vi "RT main.vi"() -> ()   [LabVIEW 2017]
doc: "This example demonstrates how to acquire a continuous amount of data (Waveform) using the DAQ device's internal clock. It also shows how to synchronize two devices for different device families (E Series, S Series, M Series, X Series, DSA, and SC Express), to simultaneously acquire the data.\n\nFor instructions on how to connect your signals to the DAQ device, refer to your device documentation."
uses:
  <vilib>/addons/_NISVFA/_Shared subVIs/Controls/svc_Engineering Units Text Ring.ctl
  <vilib>/addons/_NISVFA/_Shared subVIs/Controls/svc_Weighting Filter Text Ring.ctl
  typedefs/Data.ctl
  <vilib>/Utility/error.llb/DialogType.ctl
  <vilib>/DAQmx/read.llb/DAQmx Read (Analog 1D Wfm NChan NSamp).vi
  <vilib>/Analysis/baseanly.llb/Mean (DBL).vi
  <vilib>/DAQmx/read.llb/DAQmx Read (Analog Wfm 1Chan NSamp).vi
  <vilib>/addons/Sound and Vibration/svt_Calibration/SVL Scale Voltage to EU (1 Ch).vi
  <vilib>/DAQmx/read.llb/DAQmx Read (Analog DBL 1Chan 1Samp).vi
  <vilib>/addons/_NISVFA/_Shared subVIs/Common/svc_Set SV Channel Info.vi
  <vilib>/addons/_NISVFA/_Shared subVIs/Common/svc_Set SV Channel Info (variant).vi
  <vilib>/addons/_NISVFA/_Shared subVIs/Common/SVL Set dB Reference (variant).vi
  <vilib>/DAQmx/create/channels.llb/DAQmx Create Channel (AI-Voltage-Basic).vi
  <vilib>/DAQmx/configure/timing.llb/DAQmx Timing (Sample Clock).vi
  <vilib>/DAQmx/create/channels.llb/DAQmx Create Channel (AI-Temperature-Thermocouple).vi
  <vilib>/httpClient/POSTBuffer.vi
  <vilib>/DAQmx/miscellaneous.llb/DAQmx Fill In Error Info.vi
  <vilib>/addons/Sound and Vibration/Order Analysis/Tach Process/OAT Analog Tacho Process (1 Tacho).vi
  <vilib>/addons/_NISVFA/_Shared subVIs/Common/svc_Engineering Units to Unit Label.vi
  <vilib>/addons/_NISVFA/_Shared subVIs/Common/svc_Compute Scale Factor to Convert V to EU.vi
  <vilib>/addons/_NISVFA/_Shared subVIs/Common/svc_Compute Scale Factor to Convert C to EU.vi
  <vilib>/addons/_NISVFA/_Shared subVIs/Common/svc_Set dB ref if Pascal.vi
  <vilib>/addons/_NISVFA/_Shared subVIs/Common/svc_Caller VI Returned in Error Source.vi
  <vilib>/addons/Sound and Vibration/svt_Level/SVL Running RMS Level (1 Ch).vi
  <vilib>/addons/Sound and Vibration/svt_Calibration/SoundVib_Calibration.lvlib
  <vilib>/addons/Sound and Vibration/svt_Level/SoundVib_VibrationLevel.lvlib
  <vilib>/addons/Sound and Vibration/Order Analysis/Tach Process/SoundVib_TachProcess.lvlib
  <vilib>/Analysis/NI_AALBase.lvlib
  <vilib>/httpClient/LabVIEWHTTPClient.lvlib
  <vilib>/NI_Real-Time Target Support.lvlib
panel:
  out "dequeue elements":T1 {"RMS" format="%0.6f"; "RPM" format="%0.2f"; "Voltage" format="%0.2f"; "Current" format="%0.2f"; "Temperature" format="%0.2f"}
  out "flush elements":T1[](array[typedef]) {"RMS" format="%0.2f"; "RPM" format="%0.2f"; "Voltage" format="%0.2f"; "Current" format="%0.2f"; "Temperature" format="%0.2f"}
  out "Y":bool
  out "Numeric 2":i32
  out "Numeric":i32
  out "# elements in queue":i32
  in  "DIO STOP":bool
  in  "Buttoon 1":bool
  in  "Button 2":bool
  in  "Button 3":bool
  in  "Ipad 2":bool
  in  "Ipad 3":bool
  in  "Ipad 1":bool
  out "Valve":bool[](array[boolean])
  in  "Web server LED":bool
  out "X":bool
  out "JSON":string
  in  "integration time [s]":dbl=1.0
  out "Temp.":dbl format="%0.2f"
  out "Current":dbl format="%0.2f"
  out "Voltage":dbl format="%0.2f"
  out "RPM mean":dbl format="%0.2f"
  out "Motor Voltage & Current":waveform(dbl)[](graph)
  in  "Vibration Channel Info":T4={"sensor sensitivity"=1000.0, "engineering units"=1, "dB reference"=1.0, "custom label"="EU", "weighting filter"=0, "pregain"=0.0} {"pregain" format="%.2f"; "weighting filter" items=["Linear", "A-weighting", "B-weighting", "C-weighting", "ITU-R 468-4", "Dolby", "CCITT", "C-message", "Wb", "Wc", "Wd", "We", "Wf", "Wh", "Wj", "Wk", "Wm", "AES17 20 kHz lowpass", "AES17 40 kHz lowpass", "AES17 20 kHz highpass", "AES17 40 kHz highpass"]; "dB reference" format="%^.1e"; "engineering units" items=["custom..."=0, "V"=1, "A"=21, "C"=30, "pC"=31, "s"=32, "-"=29, "Pa"=2, "N"=20, "g"=3, "m/s^2"=4, "m/s"=5, "m"=6, "mm/s"=12, "mm"=13, "micron/s"=14, "micron"=15, "in/s^2"=7, "in/s"=8, "in"=9, "mil/s"=10, "mil"=11, "rad/s^2"=16, "rad/s"=17, "rad"=18, "deg/s^2"=26, "deg/s"=27, "deg"=28, "RPM"=22, "cycle/s^2"=23, "Hz"=24, "cycle"=25, "strain"=19]; "sensor sensitivity" format="%#_5f"}
  out "running RMS":dbl caption="g rms" format="%0.6f"
  in  "Acquire Stop":bool
  in  "CJC Channel":refnum<k21>
  in  "CJC Value":dbl=25.0 format="%0.2f"
  in  "CJC Source":i32(ring)=10116 items=["Built-In"=10200, "Constant Value"=10116, "Channel"=10113]
  in  "Thermocouple Type":i32(ring)=10073 items=["J"=10072, "K"=10073, "N"=10077, "R"=10082, "S"=10085, "T"=10086, "B"=10047, "E"=10055]
  in  "Units":i32(ring)=10143 items=["Deg C"=10143, "Deg F"=10144, "Kelvins"=10325, "Deg R"=10145, "From Custom Scale"=10065]
  in  "Max Temperature":dbl=35.0
  in  "Min Temperature":dbl
  out "Thermocouple waveform":dbl(graph)
  in  "Thermocouple Sample":i32=1
  in  "Motor Voltage & \nCurrent & RPM Sample":i32=2560
  in  "Motor Voltage & Current & RPM Sample Rate":dbl=25600.0
  in  "Thermocouple":tag="Mod3/ai0"
  out "Vibration":waveform(dbl)(graph)
  in  "Vibration Sample":i32=2560
  in  "Vibration Sample Rate":dbl=25600.0
  in  "Motor Voltage &Current& RPM":tag="Mod2/ai0:2"
  in  "Vibration":tag="Mod1/ai0"
  # "Vibration Settings"
  # "Vibration"
  # "Motor Voltage & Current & RPM"
  # "Motor Voltage & current & RPM Settings"
  # "Temperature"
  # "Tempearture"
  # "Thermocouple Settings"
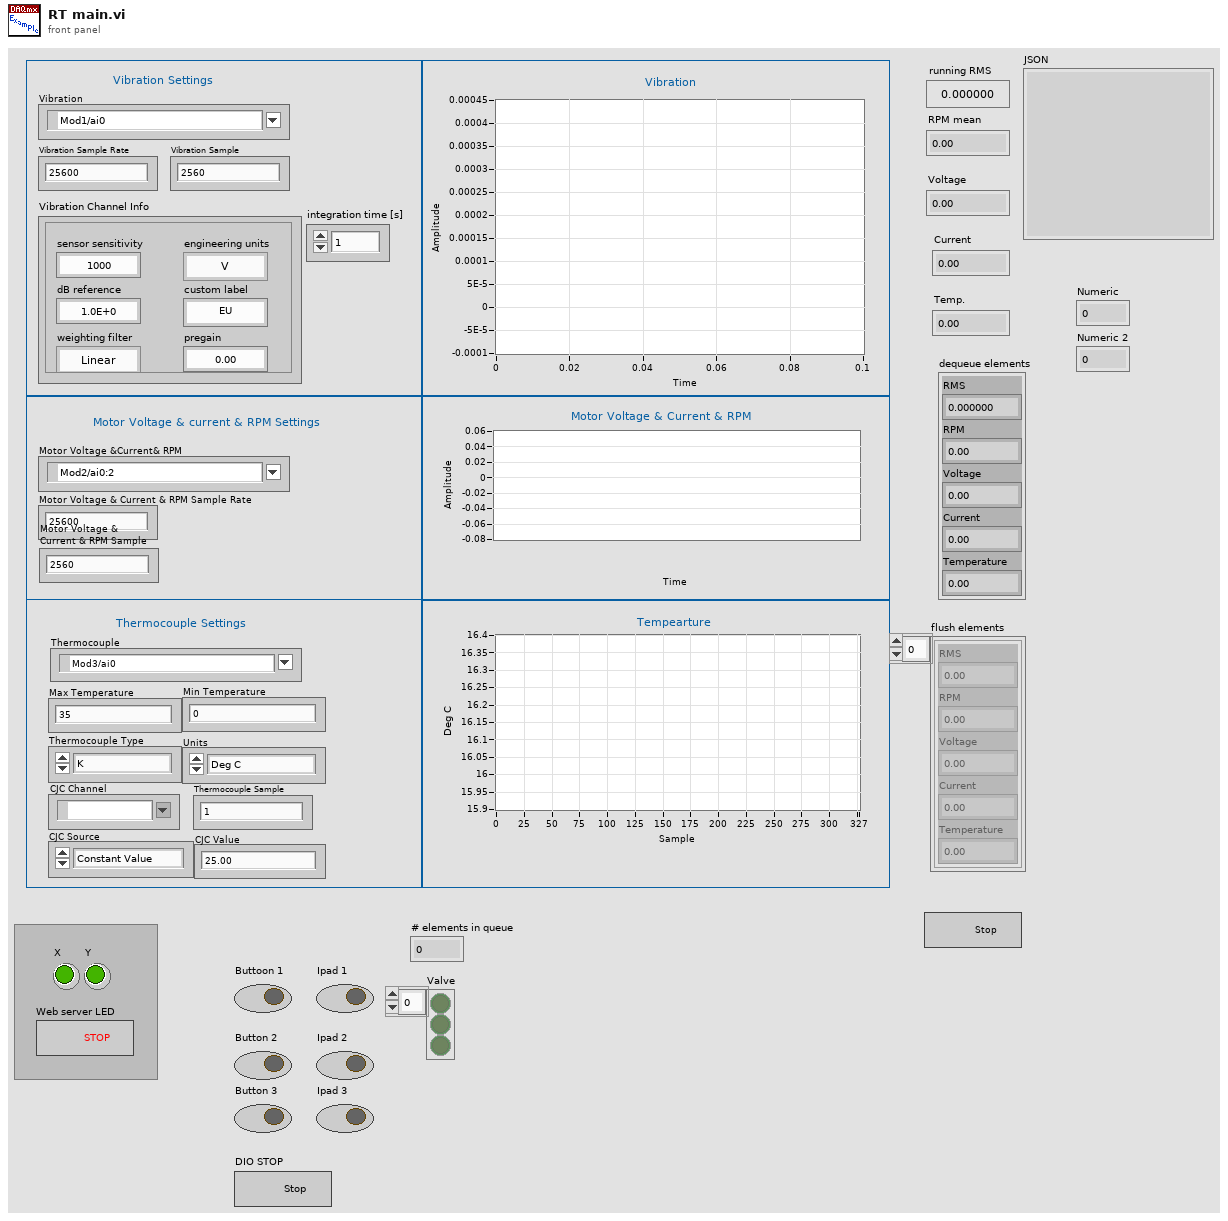
[diagram p1: front panel]
types:
  T1 = typedef "Data.ctl" = cluster{"RMS":dbl, "RPM":dbl, "Voltage":dbl, "Current":dbl, "Temperature":dbl}
  T2 = typedef "svc_Engineering Units Text Ring.ctl" = u16
  T3 = typedef "svc_Weighting Filter Text Ring.ctl" = u16
  T4 = cluster{"sensor sensitivity":dbl, "engineering units":T2, "dB reference":dbl, "custom label":string, "weighting filter":T3, "pregain":dbl}
  T5 = typedef "DialogType.ctl" = u16
  T6 = typedef "SoundVib_TachProcess.lvlib/speed profile.ctl" = cluster{"time [s]":dbl[], "speed [RPM]":dbl[]}
  T7 = typedef "LabVIEWHTTPClient.lvlib/ClientHandle.ctl" = refnum<k1>
  T8 = cluster{"RMS":dbl, "RPM":dbl, "Voltage":dbl, "Current":dbl, "Temperature":dbl}
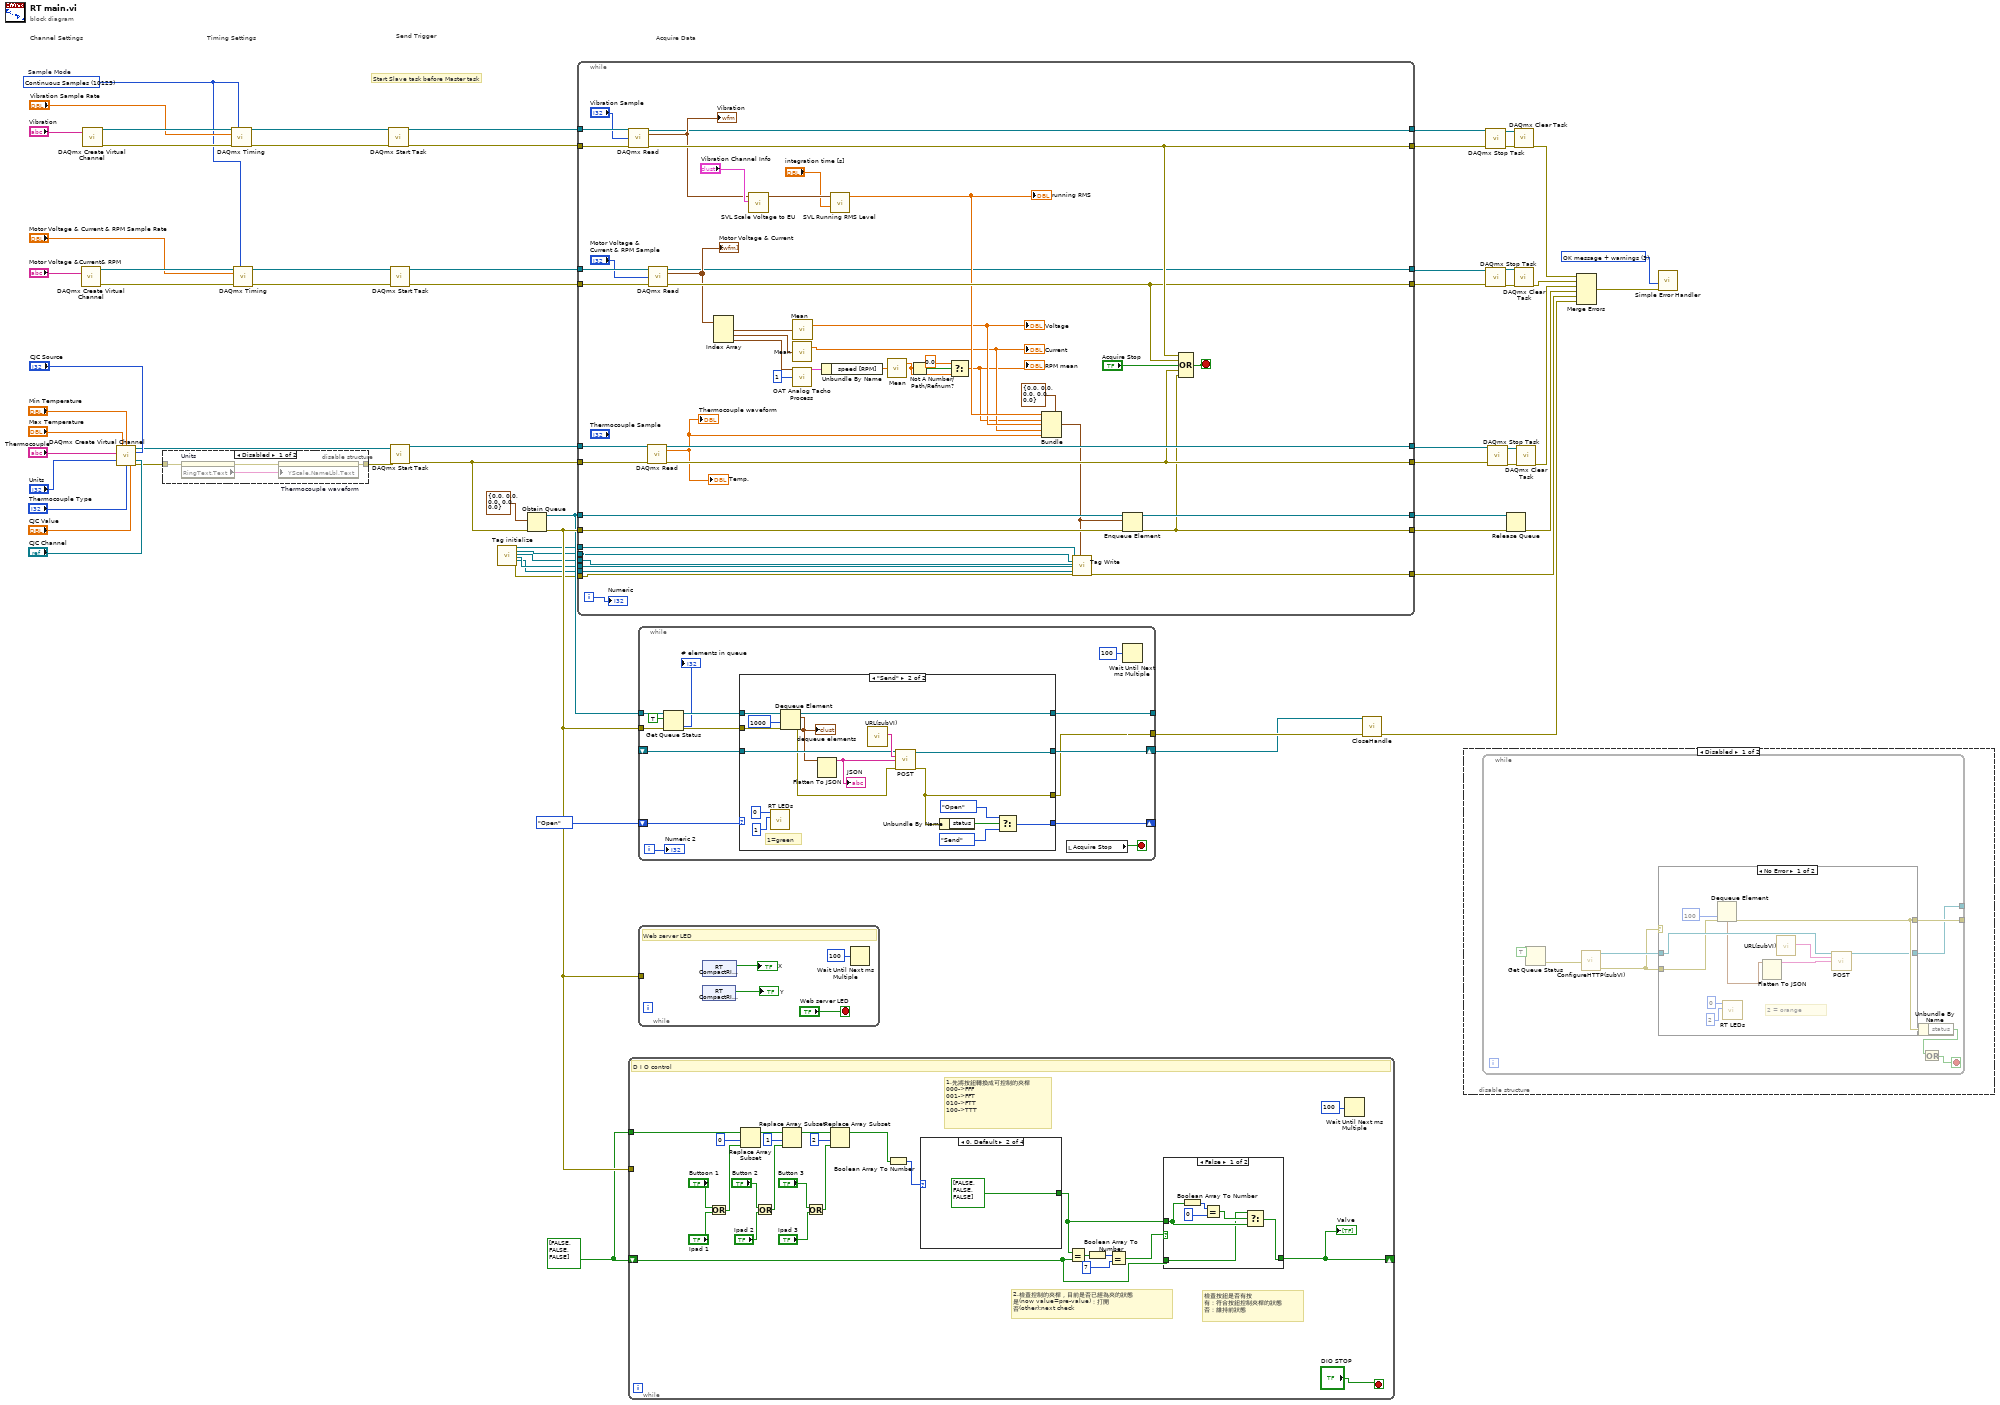
[diagram p0: block diagram]
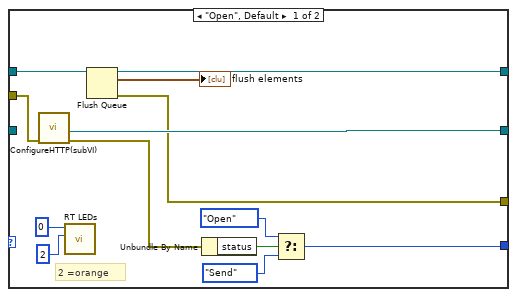
[diagram p3: hidden frame]
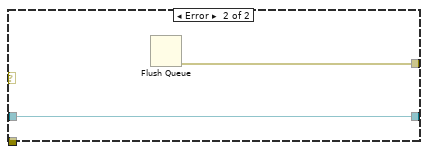
[diagram p4: hidden frame]
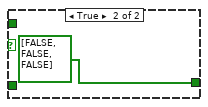
[diagram p6: hidden frame]
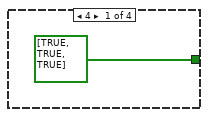
[diagram p7: hidden frame]
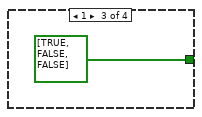
[diagram p8: hidden frame]
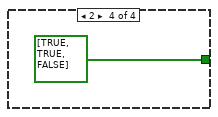
[diagram p9: hidden frame]
diagram:
  w9 = bool[] [FALSE, FALSE, FALSE]
  w41 = T5 3 items=["no dialog", "OK message", "continue or stop message", "OK message + warnings", "continue/stop + warnings"] ("type of dialog (OK msg:1)")
  w40 = 10123 items=["Finite Samples"=10178, "Continuous Samples"=10123, "Hardware Timed Single Point"=12522]  # Sample Mode
  # "Send Trigger"
  # "Acquire Data"
  # "Timing Settings"
  # "Channel Settings"
  # "Start Slave task before Master task"
  n1 = call-poly <vilib>:"DAQmx Create Virtual Channel.vi"("physical channels"="Motor Voltage &Current& RPM") -> ("task out"=w44:refnum<k21>, "error out"=w46:errorcluster)  [unwired: 13 in]
  n2 = call-poly <vilib>:"DAQmx Create Virtual Channel.vi"("physical channels"="Vibration") -> ("task out"=w48:refnum<k21>, "error out"=w47:errorcluster)  [unwired: 13 in]
  n3 = call-poly <vilib>:"DAQmx Create Virtual Channel.vi"("maximum value"="Max Temperature", "minimum value"="Min Temperature", "physical channels"="Thermocouple", "cjc source"="CJC Source", "units"="Units", "cjc channel"="CJC Channel", "thermocouple type"="Thermocouple Type", "cjc value"="CJC Value") -> ("task out"=w22:refnum<k21>, "error out"=w24:errorcluster)  [unwired: 6 in]
  n4 = disable-structure shown="Disabled" {
    disable-tunnel: w24 -> [w69 w70]
    disable-tunnel: [w66 w70] -> w21
    frame Disabled {
      n5 = property on="Units" class="Ring (strict)"(error in=w69) -> (error out=w67:errorcluster, "RingText.Text"=w68:string)  [unwired: 1 in, 1 out]
      n6 = property on="Thermocouple waveform" class="WFChart (strict)"(error in=w67, "YScale.NameLbl.Text"=w68) -> (error out=w66:errorcluster)  [unwired: 1 in, 1 out]
    }
    frame Enabled {
    }
  }
  n7 = call-poly <vilib>:"DAQmx Timing.vi"("task/channels in"=w48, "sample mode"=w40, "rate"="Vibration Sample Rate", "error in"=w47) -> ("task out"=w17:refnum<k21>, "error out"=w38:errorcluster)  [unwired: 10 in]
  n8 = call-poly <vilib>:"DAQmx Timing.vi"("task/channels in"=w44, "sample mode"=w40, "rate"="Motor Voltage & Current & RPM Sample Rate", "error in"=w46) -> ("task out"=w45:refnum<k21>, "error out"=w43:errorcluster)  [unwired: 10 in]
  n9 = call <vilib>:"DAQmx Start Task.vi"("task/channels in"=w17, "error in"=w38) -> ("task out"=w65:refnum<k21>, "error out"=w64:errorcluster)  [unwired: 12 in]
  n10 = call <vilib>:"DAQmx Start Task.vi"("task/channels in"=w45, "error in"=w43) -> ("task out"=w63:refnum<k21>, "error out"=w62:errorcluster)  [unwired: 12 in]
  n11 = call <vilib>:"DAQmx Start Task.vi"("task/channels in"=w22, "error in"=w21) -> ("task out"=w37:refnum<k21>, "error out"=w16:errorcluster)  [unwired: 12 in]
  n12 = call "Tag initialize.vi"() -> ("RMS tag"=w7:refnum<class "NI Skyline Tag.lvclass">, "RPM tag"=w6:refnum<class "NI Skyline Tag.lvclass">, "Voltage tag"=w5:refnum<class "NI Skyline Tag.lvclass">, "Current Tag"=w4:refnum<class "NI Skyline Tag.lvclass">, "Temper tag"=w3:refnum<class "NI Skyline Tag.lvclass">, "error out"=w2:errorcluster)  [unwired: 14 in]
  n13 = Obtain Queue(element data type=T1 {"RMS"=0.0, "RPM"=0.0, "Voltage"=0.0, "Current"=0.0, "Temperature"=0.0} ("Data"), error in (no error)=w16) -> (queue out=w12:refnum<queue>, error out=w13:errorcluster)  [unwired: 3 in, 1 out]
  n14 = while {
    tunnel: w37 -> [w111]
    tunnel: w16 -> [w110]
    tunnel: [w109] -> w34
    tunnel: [w108] -> w33
    tunnel: w12 -> [w99]
    tunnel: [w96] -> w20
    tunnel: [w95] -> w19
    tunnel: w13 -> [w94]
    tunnel: w65 -> [w118]
    tunnel: [w87] -> w61
    tunnel: w63 -> [w115]
    tunnel: [w88] -> w57
    tunnel: w62 -> [w114]
    tunnel: [w113] -> w56
    tunnel: w64 -> [w117]
    tunnel: [w116] -> w60
    tunnel: w7 -> [w77]
    tunnel: w6 -> [w76]
    tunnel: w5 -> [w75]
    tunnel: w4 -> [w74]
    tunnel: w3 -> [w73]
    tunnel: w2 -> [w72]
    tunnel: [w71] -> w1
    i -> [w86]
    stop <- w119 stop-if-true
    n15 = call-poly <vilib>:"DAQmx Read.vi"("task/channels in"=w118, "number of samples per channel"="Vibration Sample", "error in"=w117) -> ("task out"=w87:refnum<k21>, "data"=w90:waveform(dbl), "error out"=w116:errorcluster)  [unwired: 10 in]
    "Vibration" <- w90
    n16 = call-poly <vilib>:"DAQmx Read.vi"("task/channels in"=w111, "error in"=w110) -> ("task out"=w109:refnum<k21>, "data"=w93:dbl, "error out"=w108:errorcluster)  [unwired: 11 in]
    "Thermocouple waveform" <- w93
    "Temp." <- w93
    n17 = call-poly <vilib>:"DAQmx Read.vi"("task/channels in"=w115, "number of samples per channel"="Motor Voltage & \nCurrent & RPM Sample", "error in"=w114) -> ("task out"=w88:refnum<k21>, "data"=w101:waveform(dbl)[], "error out"=w113:errorcluster)  [unwired: 10 in]
    "Motor Voltage & Current" <- w101
    n18 = Index Array(array=w101) -> (element #1=w100:waveform(dbl), element #2=w92:waveform(dbl), element #3=w91:waveform(dbl))  [unwired: 3 in]
    n19 = call-poly <vilib>:"SVL Scale Voltage to EU.vi"("channel info"="Vibration Channel Info", "signal [V]"=w90) -> ("scaled signal [EU]"=w105:waveform(dbl))  [unwired: 7 in, 2 out]
    n20 = call-poly <vilib>:"Mean.vi"("X"=w92) -> ("mean"=w83:dbl)  [unwired: 1 out]
    "Current" <- w83
    n21 = call-poly <vilib>:"OAT Analog Tacho Process.vi"("analog tacho signal"=w91, "pulse/revolution (1)"=1) -> ("speed profile"=w103:T6)  [unwired: 9 in, 4 out]
    n22 = call-poly <vilib>:"Mean.vi"("X"=w100) -> ("mean"=w97:dbl)  [unwired: 1 out]
    "Voltage" <- w97
    n23 = Unbundle By Name(w103) -> ("speed [RPM]"=w102:dbl[])
    n24 = call-poly <vilib>:"SVL Running RMS Level.vi"("integration time [s]"="integration time [s]", "scaled signal [EU]"=w105) -> ("running RMS level [EU rms]"=w98:dbl)  [unwired: 6 in, 3 out]
    "running RMS" <- w98
    n25 = call-poly <vilib>:"Mean.vi"("X"=w102) -> ("mean"=w79:dbl)  [unwired: 1 out]
    n26 = Not A Number/Path/Refnum?(number/path/refnum=w79) -> (NaN/Path/Refnum?=w82:bool)
    n27 = Select(t=0.0, s=w82, f=w79) -> (s? t:f=w80:dbl)
    "RPM mean" <- w80
    n28 = Bundle(cluster=T1 {"RMS"=0.0, "RPM"=0.0, "Voltage"=0.0, "Current"=0.0, "Temperature"=0.0} ("Data"), "RMS"=w98, "RPM"=w80, "Voltage"=w97, "Current"=w83, "Temperature"=w93) -> (w78:T1)
    n29 = call "Tag Write.vi"("RMS tag"=w77, "RPM tag"=w76, "Voltage tag"=w75, "Current tag"=w74, "Temper tag"=w73, "error in (no error)"=w72, "Data"=w78) -> ("error out"=w71:errorcluster)  [unwired: 12 in]
    n30 = Enqueue Element(queue=w99, element=w78, error in (no error)=w94) -> (queue out=w96:refnum<queue>, error out=w95:errorcluster)  [unwired: 1 in, 1 out]
    n31 = Compound Arithmetic op=OR(w116, w113, "Acquire Stop", w108, w95) -> (w119:bool)
    "Numeric" <- w86
  }
  n32 = while {
    shift-right: [w121] -> _
    shift-left: w9 -> [w122]
    tunnel: w13 -> [_]
    tunnel: w9 -> [w120]
    stop <- "DIO STOP" stop-if-true
    # "1.先將按鈕轉換成可控制的夾桿\n000->FFF\n001->FFT\n010->FTT\n100->TTT"
    # "檢查按鈕是否有按\n有：符合按鈕控制夾桿的狀態\n否：維持前狀態"
    # "2.檢查控制的夾桿，目前是否已經為夾的狀態\n是(now value=pre-value)：打開\n否(other):next check"
    # "D I O control"
    n33 = Or(x="Buttoon 1", y="Ipad 1") -> (x .or. y?=w137:bool)
    n34 = Replace Array Subset(array=w120, new element=w137, index=0) -> (w144:bool[])
    n35 = Or(x="Button 2", y="Ipad 2") -> (x .or. y?=w131:bool)
    n36 = Replace Array Subset(array=w144, new element=w131, index=1) -> (w143:bool[])
    n37 = Or(x="Button 3", y="Ipad 3") -> (x .or. y?=w130:bool)
    n38 = Replace Array Subset(array=w143, new element=w130, index=2) -> (w123:bool[])
    n39 = Boolean Array To Number(Boolean array=w123) -> (number=w125:u32)
    n40 = case shown="0, Default" w125 {
      tunnel: [bool[] [TRUE, TRUE, TRUE] ("Button") bool[] [FALSE, FALSE, FALSE] ("Button") bool[] [TRUE, FALSE, FALSE] ("Button") bool[] [TRUE, TRUE, FALSE] ("Button")] -> w129
      frame 4 {
      }
      frame 0, Default {
      }
      frame 1 {
      }
      frame 2 {
      }
    }
    n41 = Equal?(x=w129, y=w122) -> (x = y?=w126:bool[])
    n42 = Boolean Array To Number(Boolean array=w126) -> (number=w127:u32)
    n43 = Equal?(x=w127, y=u32 7) -> (x = y?=w128:bool)
    n44 = case shown="False" w128 {
      tunnel: [w146 bool[] [FALSE, FALSE, FALSE] ("Button")] -> w121
      tunnel: w129 -> [w148 _]
      tunnel: w122 -> [w147 _]
      frame False {
        n45 = Boolean Array To Number(Boolean array=w148) -> (number=w150:u32)
        n46 = Equal?(x=w150, y=u32 0) -> (x = y?=w149:bool)
        n47 = Select(t=w147, s=w149, f=w148) -> (s? t:f=w146:bool[])
      }
      frame True {
      }
    }
    "Valve" <- w121
    n48 = Wait Until Next ms Multiple(millisecond multiple=u32 100) -> ()  [unwired: 1 out]
  }
  n49 = while {
    shift-right: [w170] -> _
    shift-left: enum16{"Open", "Send"}."Open" -> [w171]
    shift-right: [w166] -> w14
    shift-left: _ -> [w165]
    tunnel: [w163] -> w15
    tunnel: w13 -> [w162]
    tunnel: w12 -> [w161]
    tunnel: [w167] -> _
    i -> [w158]
    stop <- w164 stop-if-true
    n50 = Get Queue Status(queue=w161, return elements? (F)=TRUE, error in (no error)=w162) -> (queue out=w168:refnum<queue>, error out=w169:errorcluster, # elements in queue=→"# elements in queue":i32)  [unwired: 5 out]
    n51 = case shown="\"Send\"" w171 {
      tunnel: [w181 w200] -> w170
      tunnel: w169 -> [w180 w196]
      tunnel: w168 -> [w179 w197]
      tunnel: [w178 w192] -> w167
      tunnel: [w175 w193] -> w166
      tunnel: w165 -> [_ w194]
      tunnel: [w173 w188] -> w163
      frame "Open", Default {
        # "2 =orange"
        n52 = call "ConfigureHTTP(subVI).vi"("error in (no error)"=w180) -> ("error out"=w174:errorcluster, "Refnum out"=w175:T7)  [unwired: 9 in]
        n53 = call <vilib>:"RT LEDs.vi"("State"=2, "LED Num"=0) -> ()  [unwired: 4 in, 2 out]
        n54 = Flush Queue(queue=w179) -> (queue out=w178:refnum<queue>, remaining elements=→"flush elements":T1[], error out=w173:errorcluster)  [unwired: 1 in]
        n55 = Unbundle By Name(w174) -> ("status"=w184:bool)
        n56 = Select(t=enum16{"Open", "Send"}."Open", s=w184, f=enum16{"Open", "Send"}."Send") -> (s? t:f=w181:enum16{"Open", "Send"})
      }
      frame "Send" {
        # "1=green"
        n57 = call <vilib>:"RT LEDs.vi"("State"=1, "LED Num"=0) -> ()  [unwired: 4 in, 2 out]
        n58 = Dequeue Element(queue=w197, timeout in ms (-1)=1000, error in (no error)=w196) -> (queue out=w192:refnum<queue>, element=w187:T1, error out=w189:errorcluster)  [unwired: 1 out]
        "dequeue elements" <- w187
        n59 = Flatten To JSON(anything=w187) -> (JSON string=w186:string)  [unwired: 2 in, 1 out]
        "JSON" <- w186
        n60 = call "URL(subVI).vi"() -> ("URL"=w195:string)  [unwired: 11 in]
        n61 = call-poly <vilib>:"POST.vi"("client handle"=w194, "url"=w195, "buffer"=w186, "error in (no error)"=w189) -> ("client handle out"=w193:T7, "error out"=w188:errorcluster)  [unwired: 8 in, 2 out]
        n62 = Unbundle By Name(w188) -> ("status"=w201:bool)
        n63 = Select(t=enum16{"Open", "Send"}."Open", s=w201, f=enum16{"Open", "Send"}."Send") -> (s? t:f=w200:enum16{"Open", "Send"})
      }
    }
    n64 = local read "Acquire Stop"() -> (w164:bool)
    n65 = Wait Until Next ms Multiple(millisecond multiple=u32 100) -> ()  [unwired: 1 out]
    "Numeric 2" <- w158
  }
  n66 = while {
    tunnel: w13 -> [_]
    stop <- "Web server LED" stop-if-true
    # "Web server LED"
    n67 = shared-variable "RT CompactRIO Target \\variable.lvlib\\X"() -> (→"X":bool)  [unwired: 1 in, 1 out]
    n68 = shared-variable "RT CompactRIO Target \\variable.lvlib\\Y"() -> (→"Y":bool)  [unwired: 1 in, 1 out]
    n69 = Wait Until Next ms Multiple(millisecond multiple=u32 100) -> ()  [unwired: 1 out]
  }
  n70 = call <vilib>:"CloseHandle.vi"("client handle"=w14, "error in (no error)"=w15) -> ("error out"=w8:errorcluster)  [unwired: 13 in]
  n71 = disable-structure shown="Disabled" {
    frame Disabled {
      n72 = while {
        tunnel: [w211] -> _
        tunnel: [w208] -> _
        stop <- w212 stop-if-true
        n73 = Get Queue Status(return elements? (F)=TRUE) -> (error out=w210:errorcluster)  [unwired: 2 in, 7 out]
        n74 = call "ConfigureHTTP(subVI).vi"("error in (no error)"=w210) -> ("error out"=w206:errorcluster, "Refnum out"=w209:T7)  [unwired: 9 in]
        n75 = case shown="No Error" w206 {
          tunnel: [w219 w225] -> w211
          tunnel: w209 -> [w221 w224]
          tunnel: [w220 w224] -> w208
          tunnel: w206 -> [w218 _]
          frame No Error {
            # "2 = orange"
            n76 = Dequeue Element(timeout in ms (-1)=100, error in (no error)=w218) -> (element=w216:T8, error out=w219:errorcluster)  [unwired: 1 in, 2 out]
            n77 = call <vilib>:"RT LEDs.vi"("State"=2, "LED Num"=0) -> ()  [unwired: 4 in, 2 out]
            n78 = Flatten To JSON(anything=w216) -> (JSON string=w217:string)  [unwired: 2 in, 1 out]
            n79 = call "URL(subVI).vi"() -> ("URL"=w222:string)  [unwired: 11 in]
            n80 = call-poly <vilib>:"POST.vi"("client handle"=w221, "url"=w222, "buffer"=w217) -> ("client handle out"=w220:T7)  [unwired: 9 in, 3 out]
          }
          frame Error {
            n81 = Flush Queue() -> (error out=w225:errorcluster)  [unwired: 2 in, 2 out]
          }
        }
        n82 = Unbundle By Name(w211) -> ("status"=w213:bool)
        n83 = Or(x=w213) -> (x .or. y?=w212:bool)  [unwired: 1 in]
      }
    }
    frame Enabled {
    }
  }
  n84 = call <vilib>:"DAQmx Stop Task.vi"("task/channels in"=w61, "error in"=w60) -> ("task out"=w58:refnum<k21>, "error out"=w59:errorcluster)  [unwired: 12 in]
  n85 = call <vilib>:"DAQmx Stop Task.vi"("task/channels in"=w57, "error in"=w56) -> ("task out"=w54:refnum<k21>, "error out"=w55:errorcluster)  [unwired: 12 in]
  n86 = call <vilib>:"DAQmx Stop Task.vi"("task/channels in"=w34, "error in"=w33) -> ("task out"=w36:refnum<k21>, "error out"=w35:errorcluster)  [unwired: 12 in]
  n87 = Release Queue(queue=w20, error in (no error)=w19) -> (error out=w18:errorcluster)  [unwired: 1 in, 2 out]
  n88 = call <vilib>:"DAQmx Clear Task.vi"("task in"=w58, "error in"=w59) -> ("error out"=w53:errorcluster)  [unwired: 13 in]
  n89 = call <vilib>:"DAQmx Clear Task.vi"("task in"=w54, "error in"=w55) -> ("error out"=w52:errorcluster)  [unwired: 13 in]
  n90 = call <vilib>:"DAQmx Clear Task.vi"("task in"=w36, "error in"=w35) -> ("error out"=w32:errorcluster)  [unwired: 13 in]
  n91 = Merge Errors(w53, w52, w32, w18, w1, w8) -> (w51:errorcluster)
  n92 = call <vilib>:"Simple Error Handler.vi"("type of dialog (OK msg:1)"=w41, "error in (no error)"=w51) -> ()  [unwired: 3 in, 5 out]
